vi ".NET Object Stream Reader.vi"(8 "error in (no error)":errorcluster, 9 ".NET TcAdsSymbolInfo":refnum<k24>, 10 ".NET Object Stream":refnum<k24>[](array[refnum]), 11 "TwinCAT ADS in":refnum<class "TwinCAT ADS.lvclass">) -> (0 "error out":errorcluster, 1 "G Object":variant, 3 "TwinCAT ADS out":refnum<class "TwinCAT ADS.lvclass">)   [LabVIEW 2018, in "TwinCAT ADS.lvclass"]
uses:
  TwinCAT ADS.lvclass
  TwinCAT.Ads
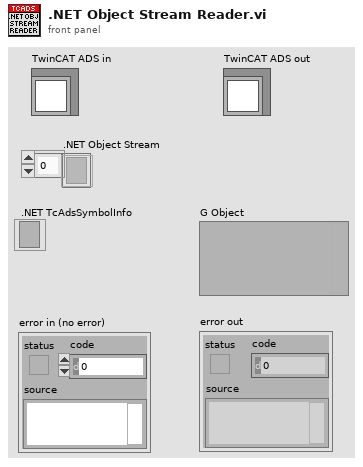
[diagram p1: front panel]
types:
  T1 = typedef "TwinCAT ADS.lvclass/Symbol Information.ctl" = cluster{"Name":string, "Short Name":string, "Size":i32, "Type Category":i32, "Type Name":string, "Type ID":i32, "Index Group":i64, "Index Offset":i64, "Child Count":i32, "Has Rpc Methods?":bool, "Comment":string}
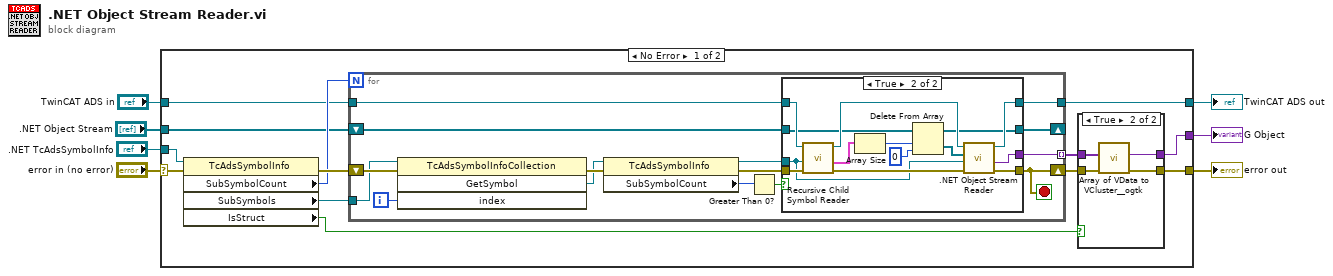
[diagram p0: block diagram]
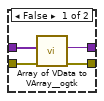
[diagram p2: hidden frame]
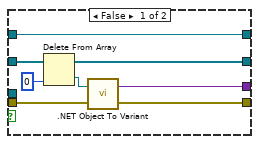
[diagram p3: hidden frame]
diagram:
  n1 = case shown="No Error" "error in (no error)" {
    selector: "error in (no error)" -> [w19 w67]
    tunnel: [w8 w67] -> w6
    tunnel: [w12 w66] -> w4
    tunnel: "TwinCAT ADS in" -> [w15 w66]
    tunnel: ".NET TcAdsSymbolInfo" -> [w20 _]
    tunnel: ".NET Object Stream" -> [w10 _]
    tunnel: [w11 _] -> w1
    frame No Error {
      n2 = property class="TcAdsSymbolInfo"(reference=w20, error in=w19) -> (error out=w18:errorcluster, "SubSymbolCount"=w17:i32, "SubSymbols"=w16:refnum<k24>, "IsStruct"=w14:bool)  [unwired: 1 out]
      n3 = for {
        N: w17 -> [_]
        tunnel: w16 -> [w29]
        tunnel: w15 -> [w38]
        tunnel: [w37] -> w13 mode=indexing
        tunnel: [w36] -> w12
        shift-right: [w32] -> w9
        shift-left: w18 -> [w43]
        shift-right: [w33] -> _
        shift-left: w10 -> [w34]
        i -> [w31]
        stop <- w32 stop-if-true
        n4 = invoke class="TcAdsSymbolInfoCollection" method="GetSymbol"(reference=w29, error in=w43, "index"=w31) -> (error out=w42:errorcluster, "GetSymbol"=w41:refnum<k24>)  [unwired: 1 in, 2 out]
        n5 = property class="TcAdsSymbolInfo"(reference=w41, error in=w42) -> (reference out=w35:refnum<k24>, error out=w39:errorcluster, "SubSymbolCount"=w30:i32)
        n6 = Greater Than 0?(x=w30) -> (x > 0?=w40:bool)
        n7 = case shown="True" w40 {
          tunnel: w39 -> [w51 w57]
          tunnel: w38 -> [w48 w65]
          tunnel: [w50 w59] -> w32
          tunnel: [w49 w58] -> w37
          tunnel: [w48 w63] -> w36
          tunnel: w35 -> [_ w52]
          tunnel: w34 -> [w47 w62]
          tunnel: [w46 w61] -> w33
          frame False {
            n8 = Delete From Array(array=w47, index=0) -> (deleted portion=w44:refnum<k24>, array with subset deleted=w46:refnum<k24>[])  [unwired: 1 in]
            n9 = call <vilib>:".NET Object To Variant.vi"("error in (no error)"=w51, ".NET object"=w44) -> ("error out"=w50:errorcluster, "variant"=w49:variant)
          }
          frame True {
            n10 = call "Recursive Child Symbol Reader.vi"("error in (no error)"=w57, ".NET TcAdsSymbolInfo"=w52, "TwinCAT ADS in"=w65) -> ("error out"=w56:errorcluster, "Symbols Information"=w55:T1[], "TwinCAT ADS out"=w64:refnum<class "TwinCAT ADS.lvclass">)  [unwired: 6 in]
            n11 = Array Size(array=w55) -> (size(s)=w54:i32)
            n12 = Delete From Array(array=w62, length=w54, index=0) -> (deleted portion=w53:refnum<k24>[], array with subset deleted=w61:refnum<k24>[])
            n13 = call-dynamic ".NET Object Stream Reader.vi"("error in (no error)"=w56, ".NET TcAdsSymbolInfo"=w52, ".NET Object Stream"=w53, "TwinCAT ADS in"=w64) -> ("error out"=w59:errorcluster, "G Object"=w58:variant, "TwinCAT ADS out"=w63:refnum<class "TwinCAT ADS.lvclass">)  [unwired: 5 in]
          }
        }
      }
      n14 = case shown="True" w14 {
        tunnel: w13 -> [w23 w27]
        tunnel: w9 -> [w24 w28]
        tunnel: [w21 w25] -> w8
        tunnel: [w22 w26] -> w11
        frame False {
          n15 = call <userlib>:"Array of VData to VArray__ogtk.vi"("error in (no error)"=w24, "1D Array of VData"=w23) -> ("error out"=w21:errorcluster, "VArray"=w22:variant)  [unwired: 8 in]
        }
        frame True {
          n16 = call <userlib>:"Array of VData to VCluster__ogtk.vi"("error in (no error)"=w28, "Array"=w27) -> ("error out"=w25:errorcluster, "VCluster"=w26:variant)  [unwired: 8 in]
        }
      }
    }
    frame Error {
    }
  }
  "error out" <- w6
  "TwinCAT ADS out" <- w4
  "G Object" <- w1
